vi "Add CPU Overall Channels.vi"(8 "error in":errorcluster, 11 "custom device":T1 format="%.0x") -> (0 "error out":errorcluster, 3 "custom device out":T1 format="%.0x")   [LabVIEW 2027, in "System Monitor System Explorer.lvlib"]
uses:
  System Monitor System Explorer.lvlib
  <vilib>/NI VeriStand/Custom Device API/Custom Device Item Ref.ctl
  <vilib>/NI VeriStand/Custom Device API/Custom Device Channel.ctl
  <vilib>/NI VeriStand/Custom Device API/Custom Device Channel Type.ctl
  <vilib>/NI VeriStand/Custom Device API/Custom Device API.lvlib
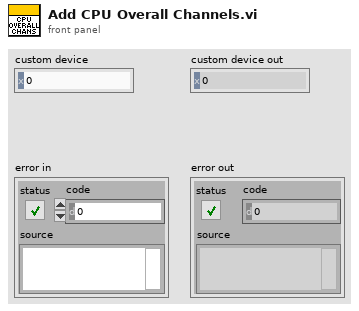
[diagram p1: front panel]
types:
  T1 = typedef "Custom Device API.lvlib/Custom Device Item Ref.ctl" = u64
  T2 = typedef "Custom Device API.lvlib/Custom Device Channel.ctl" = cluster{"Type":T3, "Units":string, "Default Value":dbl, "Faultable":bool, "Scalable":bool}
  T3 = typedef "Custom Device API.lvlib/Custom Device Channel Type.ctl" = enum16{"Input", "Output"}
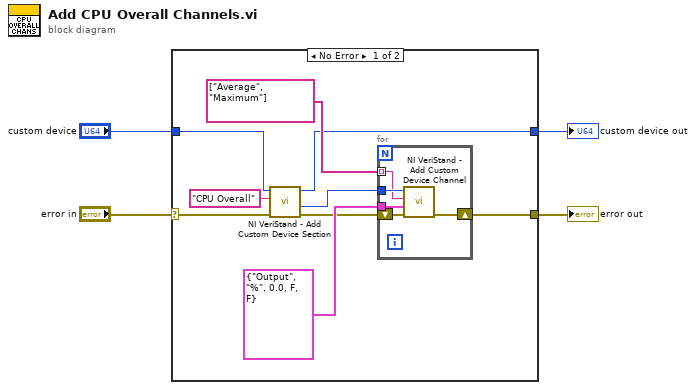
[diagram p0: block diagram]
diagram:
  n1 = case shown="No Error" "error in" {
    selector: "error in" -> [w13 w19]
    tunnel: "custom device" -> [w11 w20]
    tunnel: [w6 w20] -> w2
    tunnel: [w5 w19] -> w1
    frame No Error {
      n2 = call <vilib>:"NI VeriStand - Add Custom Device Section.vi"("error in (no error)"=w13, "Section Name"="CPU Overall", "Parent Ref in"=w11) -> ("error out"=w9:errorcluster, "Section Ptr"=w8:T1, "Parent Ref out"=w6:T1)  [unwired: 5 in, 1 out]
      n3 = for {
        tunnel: T2 {"Type"=enum."Output", "Units"="%", "Default Value"=0.0, "Faultable"=FALSE, "Scalable"=FALSE} ("Channel") -> [w18]
        tunnel: string[] ["Average", "Maximum"] -> [w15] mode=indexing
        shift-right: [w14] -> w5
        shift-left: w9 -> [w17]
        tunnel: w8 -> [w16]
        n4 = call <vilib>:"NI VeriStand - Add Custom Device Channel.vi"("error in (no error)"=w17, "Channel"=w18, "Channel Name"=w15, "Parent Ref in"=w16) -> ("error out"=w14:errorcluster)  [unwired: 4 in, 3 out]
      }
    }
    frame Error {
    }
  }
  "custom device out" <- w2
  "error out" <- w1
